vi "Write configuration.vi"(8 "error in (no error)":errorcluster, 10 "configuration":refnum<class "CEF_serializable configuration.lvclass">, 11 "Switch Instrument in":refnum<class "Switch Instrument.lvclass">) -> (0 "error out":errorcluster, 3 "Switch Instrument out":refnum<class "Switch Instrument.lvclass">)   [LabVIEW 2025, in "Switch.lvlib" / "Switch Instrument.lvclass"]
uses:
  Switch Instrument.lvclass
  Switch Instrument.lvclass/Switch Instrument.ctl
  Switch configuration/Switch configuration.lvclass
  Users/Public/Documents/Sandia National Labs/TSS Plugin/CEF.lvlibp/serializable configuration/CEF_serializable configuration.lvclass
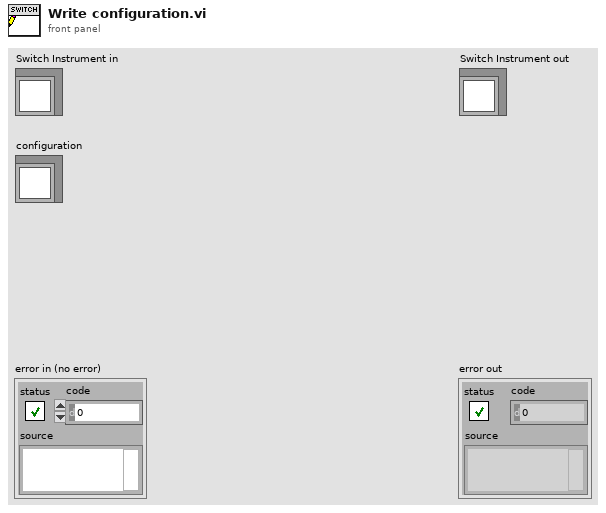
[diagram p1: front panel]
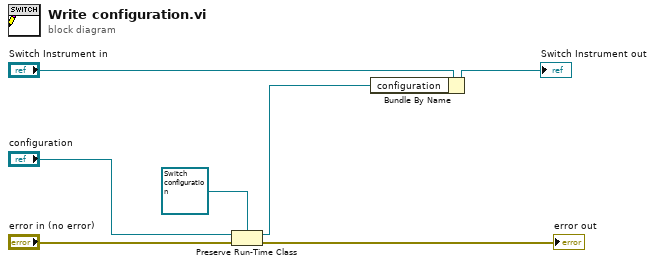
[diagram p0: block diagram]
diagram:
  n1 = Preserve Run-Time Class(object in="configuration", error in="error in (no error)", 2:refnum<class "Switch configuration.lvclass"> refnum ("Switch.lvlib:Switch config")) -> (object out=w2:refnum<class "Switch configuration.lvclass">, error out=→"error out":errorcluster)
  n2 = Bundle By Name(cluster="Switch Instrument in", "configuration"=w2) -> (→"Switch Instrument out":refnum<class "Switch Instrument.lvclass">)
